vi "Calc Force vector.vi"(2 "Pdyn ref (Pa)":sgl, 3 "Cp distribution (time averaged)":cluster{"x/c flap (sorted)":sgl[], sgl[]}[](graph)) -> (0 "Fy (N)":sgl, 1 "Fx (N)":sgl)   [LabVIEW 2015]
panel:
  in  "Area vectors, wing (sorted)":sgl[][](array[numeric])=[[-0.0029639693, -0.0012277163], [-0.002545218, -0.0019530145], [-0.0019530145, -0.002545218], [-0.0012277163, -0.0029639693], [-0.0, -0.0063614617], [0.0012277163, -0.0029639693], [0.0019530145, -0.002545218], [0.002545218, -0.0019530145], [0.0029639693, -0.0012277163], [0.0063614617, 0.0], [0.0029639693, 0.0012277163], [0.002545218, 0.0019530145], [0.0019530145, 0.002545218], [0.0012277163, 0.0029639693], [-0.0, 0.0063614617], [-0.0012277163, 0.0029639693], [-0.0019530145, 0.002545218], [-0.002545218, 0.0019530145], [-0.0029639693, 0.0012277163], [-0.0063614617, 0.0]]
  # "Paste in values from geometry prep vi and make default. Delete z column."
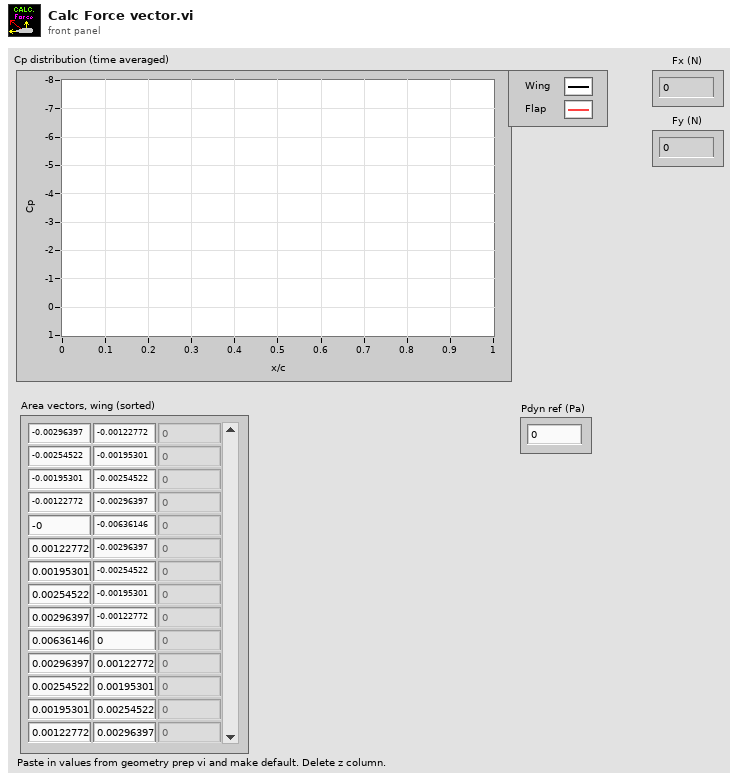
[diagram p1: front panel]
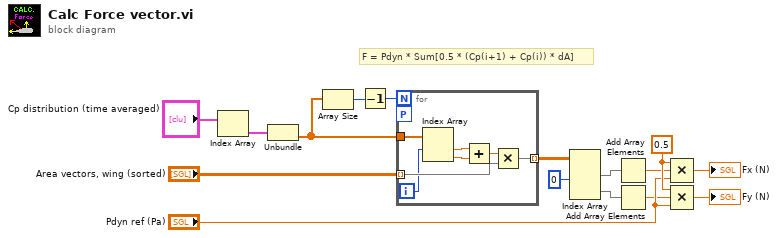
[diagram p0: block diagram]
diagram:
  w5 = sgl 0.5 ("y")
  # "F = Pdyn * Sum[0.5 * (Cp(i+1) + Cp(i)) * dA]"
  n1 = Index Array(array="Cp distribution (time averaged)") -> (element=w15:cluster{"x/c flap (sorted)":sgl[], sgl[]})  [unwired: 1 in]
  n2 = Unbundle(w15) -> (w12:sgl[])  [unwired: 1 out]
  n3 = Array Size(array=w12) -> (size(s)=w14:i32)
  n4 = Decrement(x=w14) -> (x-1=w13:i32)
  n5 = for {
    N: w13 -> [_]
    tunnel: w12 -> [w23]
    tunnel: "Area vectors, wing (sorted)" -> [w18] mode=indexing
    workers-P: _ -> [_]
    tunnel: [w20] -> w11 mode=indexing
    i -> [w17]
    n6 = Index Array(array=w23, index #1=w17) -> (element #1=w22:sgl, element #2=w21:sgl)  [unwired: 1 in]
    n7 = Add(x=w22, y=w21) -> (x+y=w19:sgl)
    n8 = Multiply(x=w19, y=w18) -> (x*y=w20:sgl[])
  }
  n9 = Index Array(array=w11, index (col) #1=0 ("disabled index (col)")) -> (element #1=w8:sgl[], element #2=w7:sgl[])  [unwired: 3 in]
  n10 = Add Array Elements(numeric array=w8) -> (sum=w2:sgl)
  n11 = Add Array Elements(numeric array=w7) -> (sum=w1:sgl)
  n12 = Compound Arithmetic op=MULTIPLY(w5, w2, "Pdyn ref (Pa)") -> (→"Fx (N)":sgl)
  n13 = Compound Arithmetic op=MULTIPLY(w5, w1, "Pdyn ref (Pa)") -> (→"Fy (N)":sgl)
